vi "test Delete Endpoint String First.vi"(8 "error in (no error)":errorcluster, 11 "TestCase in":refnum<class "Routing and Faulting Aliases Unit Tests.lvclass">) -> (0 "error out":errorcluster, 3 "TestCase out":refnum<class "Routing and Faulting Aliases Unit Tests.lvclass">)   [LabVIEW 2017, in "Routing and Faulting Aliases Unit Tests.lvclass"]
uses:
  Routing and Faulting Aliases Unit Tests.lvclass
  System Explorer/Alias.ctl
  System Explorer/Endpoint.ctl
  Shared/Alias Mapping.ctl
  Routing and Faulting Aliases Unit Tests.lvclass/Routing and Faulting Aliases Unit Tests.ctl
  <vilib>/addons/_JKI Toolkits/VI Tester/TestCase.llb/TestCase.lvclass
  System Explorer/Routing and Faulting System Explorer.lvlib
  Scripting/Routing and Faulting Scripting.lvlib
  Shared/Routing and Faulting Shared.lvlib
  C:/Program Files (x86)/National Instruments/LabVIEW 2017/vi.lib/addons/_JKI Toolkits/VI Tester/TestCase.llb/TestCase.lvclass
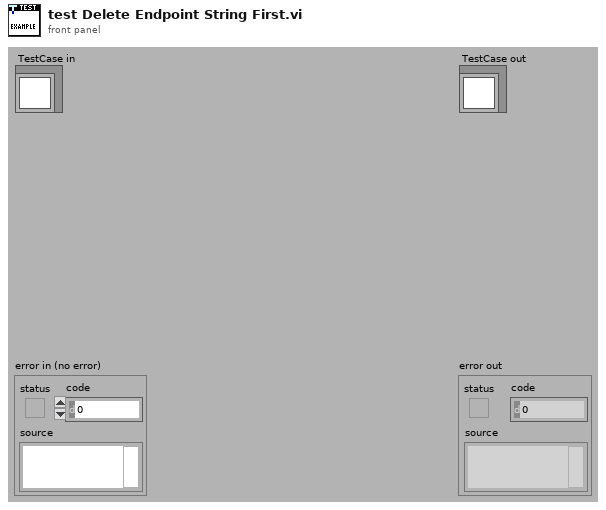
[diagram p1: front panel]
types:
  T1 = typedef "Routing and Faulting Shared.lvlib/Alias Mapping.ctl" = cluster{"Endpoint":string, "Alias":string}
  T2 = typedef "Routing and Faulting System Explorer.lvlib/Endpoint.ctl" = string
  T3 = typedef "Routing and Faulting System Explorer.lvlib/Alias.ctl" = cluster{"Endpoint":T2, "Alias":string, "Remove":bool}
  T4 = typedef "Custom Device API.lvlib/Custom Device Item Ref.ctl" = u64
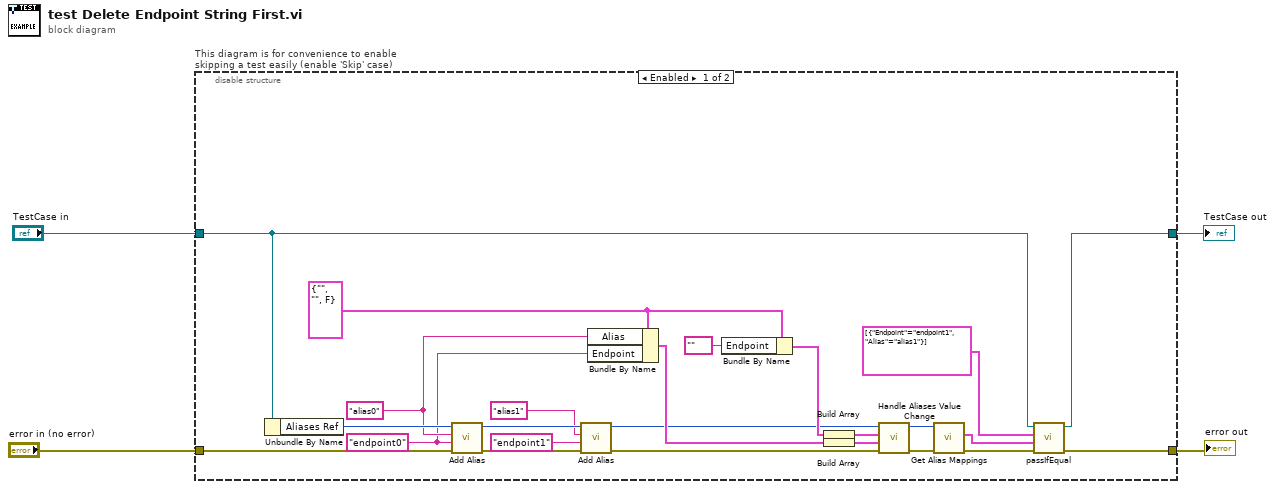
[diagram p0: block diagram]
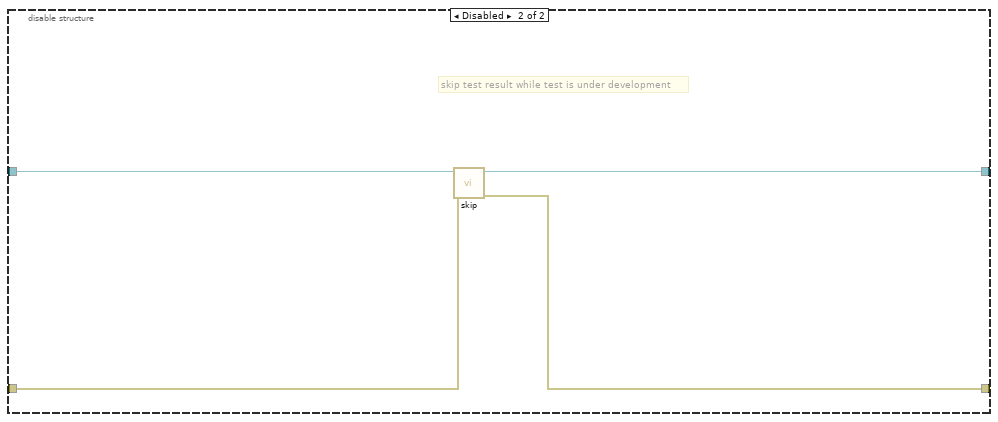
[diagram p2: hidden frame]
diagram:
  n1 = disable-structure "This diagram is for convenience to enable skipping a test easily (enable 'Skip' case)" shown="Enabled" {
    disable-tunnel: "TestCase in" -> [w24 w32]
    disable-tunnel: [w23 w30] -> w1
    disable-tunnel: [w25 w31] -> w3
    disable-tunnel: "error in (no error)" -> [w21 w29]
    frame Enabled {
      w18 = T3 {"Endpoint"="", "Alias"="", "Remove"=FALSE} ("Alias")
      w19 = "endpoint0" ("Endpoint")
      w20 = "alias0" ("Alias")
      n2 = Unbundle By Name(w24) -> ("Aliases Ref"=w22:T4)
      n3 = call "Add Alias.vi"("error in (no error)"=w21, "Endpoint"=w19, "Alias"=w20, "Endpoint Aliases Ref in"=w22) -> ("error out"=w12:errorcluster, "Endpoint Aliases Ref out"=w11:T4)  [unwired: 6 in]
      n4 = call "Add Alias.vi"("error in (no error)"=w12, "Endpoint"="endpoint1", "Alias"="alias1", "Endpoint Aliases Ref in"=w11) -> ("error out"=w8:errorcluster, "Endpoint Aliases Ref out"=w7:T4)  [unwired: 6 in]
      n5 = Bundle By Name(cluster=w18, "Alias"=w20, "Endpoint"=w19) -> (w15:T3)
      n6 = Bundle By Name(cluster=w18, "Endpoint"=T2 "") -> (w16:T3)
      n7 = Build Array(w16) -> (w14:T3[])
      n8 = Build Array(w15) -> (w13:T3[])
      n9 = call "Handle Aliases Value Change.vi"("error in (no error)"=w8, "OldVal"=w13, "NewVal"=w14, "Aliases Ref in"=w7) -> ("error out"=w28:errorcluster, "Aliases Ref out"=w27:T4)  [unwired: 6 in]
      n10 = call "Get Alias Mappings.vi"("error in (no error)"=w28, "Endpoint Aliases Ref in"=w27) -> ("error out"=w26:errorcluster, "Alias Mappings"=w6:T1[])  [unwired: 7 in, 1 out]
      n11 = call-dynamic "passIfEqual.vi"("error in (no error)"=w26, "y"=w6, "x"=T1[] [{"Endpoint"="endpoint1", "Alias"="alias1"}] ("Alias Mappings"), "TestCase in"=w24) -> ("error out"=w25:errorcluster, "TestCase out"=w23:refnum<class "Routing and Faulting Aliases Unit Tests.lvclass">)  [unwired: 6 in]
    }
    frame Disabled {
      # "skip test result while test is under development"
      n12 = call <vilib>:"skip.vi"("error in (no error)"=w29, "TestCase in"=w32) -> ("error out"=w31:errorcluster, "TestCase out"=w30:refnum<class "Routing and Faulting Aliases Unit Tests.lvclass">)  [unwired: 8 in]
    }
  }
  "error out" <- w3
  "TestCase out" <- w1
